vi "Calculate Next Position.vi"(10 "Position In":cluster{"X":i64, "Y":i64}, 11 "Velocity In":cluster{"X":i64, "Y":i64}) -> (2 "Position Out":cluster{"X":i64, "Y":i64}, 3 "Velocity Out":cluster{"X":i64, "Y":i64})   [LabVIEW 2021]
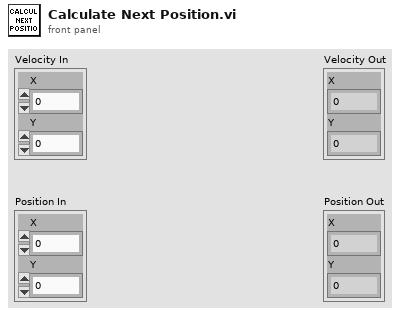
[diagram p1: front panel]
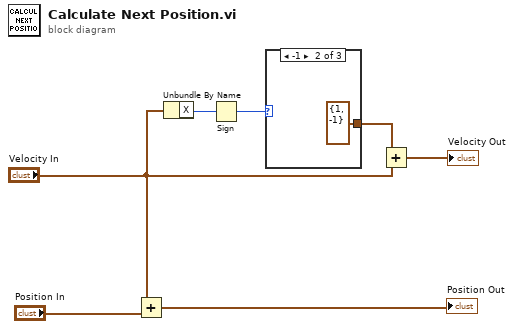
[diagram p0: block diagram]
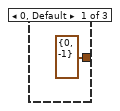
[diagram p2: hidden frame]
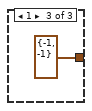
[diagram p3: hidden frame]
diagram:
  n1 = Add(x="Velocity In", y="Position In") -> (x+y=→"Position Out":cluster{"X":i64, "Y":i64})
  n2 = Unbundle By Name("Velocity In") -> ("X"=w5:i64)
  n3 = Sign(1:w5) -> (0:w4:i64)
  n4 = case shown="-1" w4 {
    tunnel: [cluster{"X":i64, "Y":i64} {"X"=0, "Y"=-1} ("Velocity In") cluster{"X":i64, "Y":i64} {"X"=1, "Y"=-1} ("Velocity In") cluster{"X":i64, "Y":i64} {"X"=-1, "Y"=-1} ("Velocity In")] -> w3
    frame 0, Default {
    }
    frame -1 {
    }
    frame 1 {
    }
  }
  n5 = Add(x=w3, y="Velocity In") -> (x+y=→"Velocity Out":cluster{"X":i64, "Y":i64})
